vi "Occupancy Grid Drawing.vi"() -> ()   [LabVIEW 2014]
panel:
  out "Occupancy Grid Drawing":dbl[][](graph)
  out "Output Occupancy Grid":dbl[][](array[numeric])
  out "Intermediate Value Array":dbl[][](array[numeric])
  in  "Particle Points":dbl[][](array[numeric])
  # "CM(X), CM(Y), Left X, Right X"
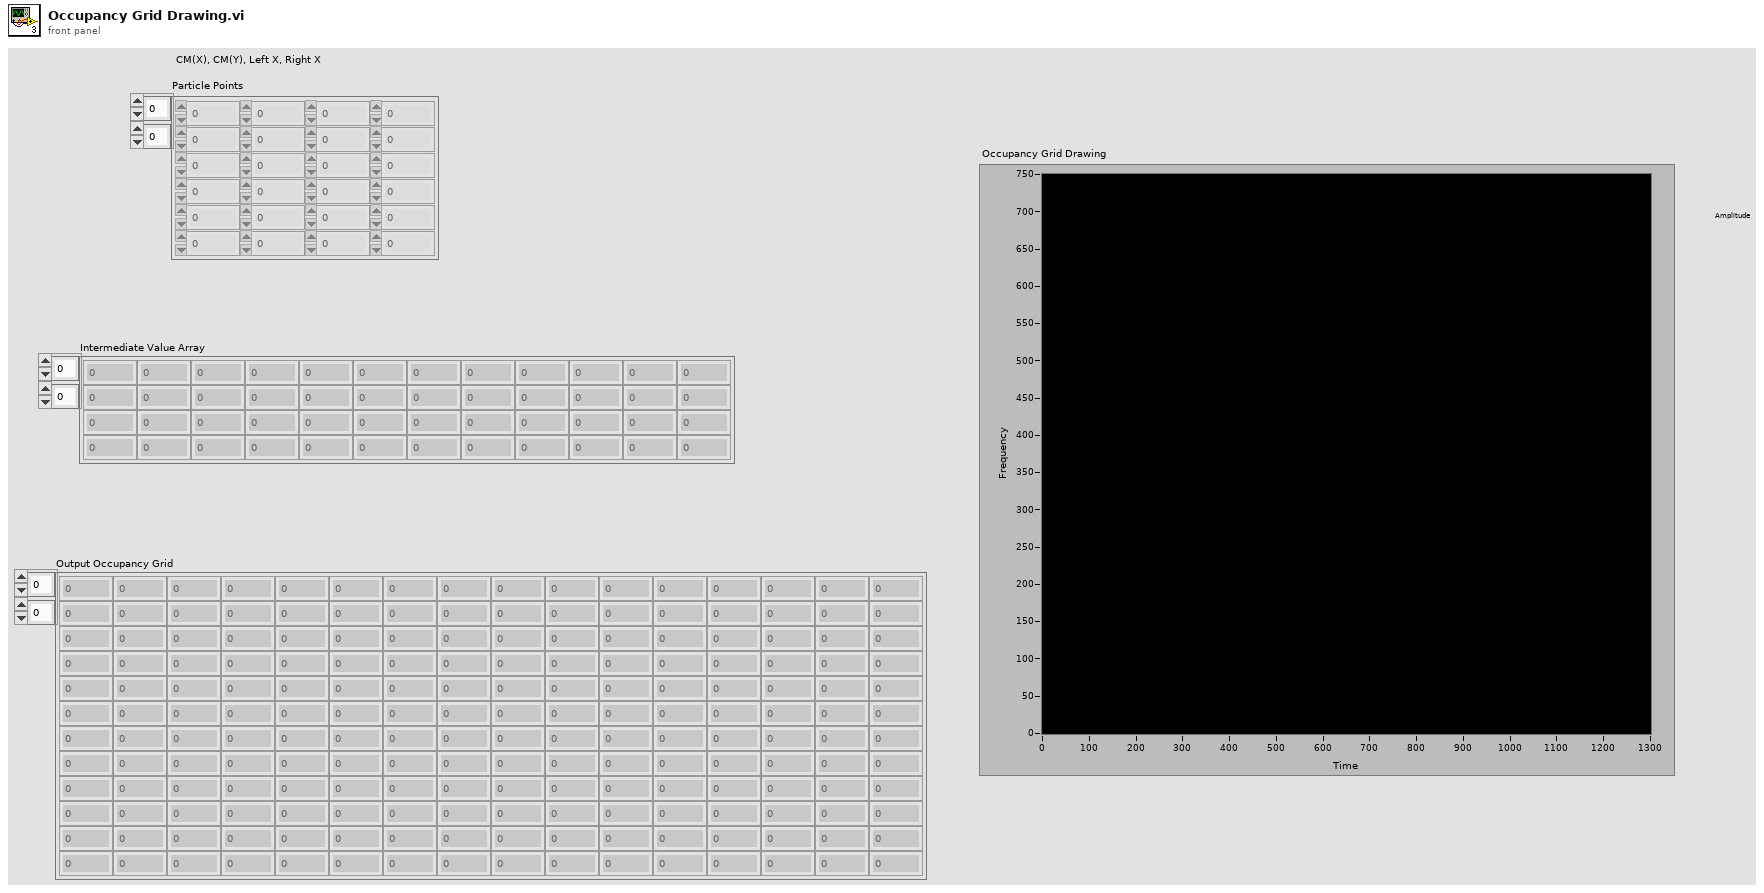
[diagram p1: front panel]
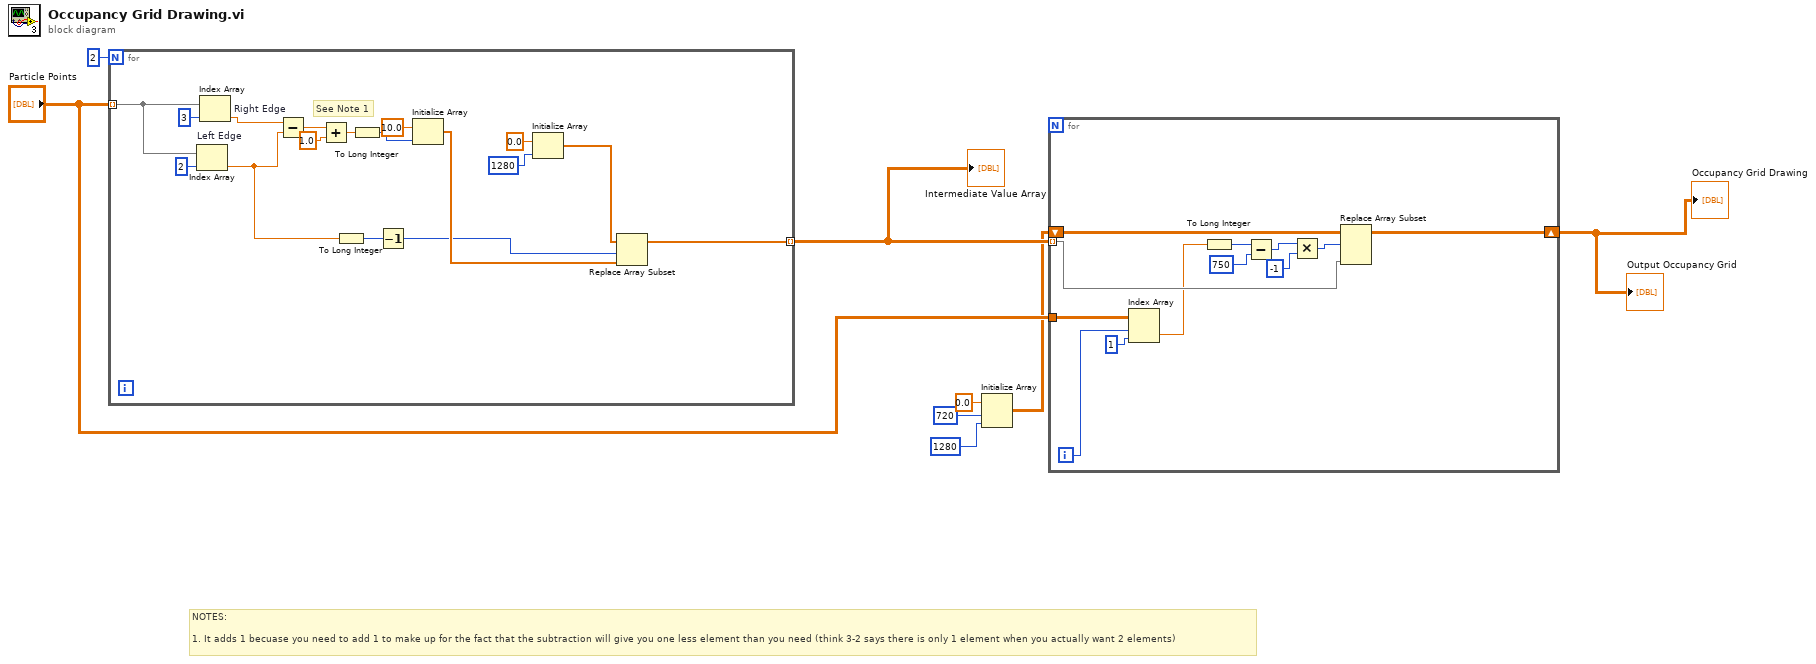
[diagram p0: block diagram]
diagram:
  # "NOTES:\n\n1. It adds 1 becuase you need to add 1 to make up for the fact that the subtraction will give you one less element than you need (think 3-2 says there is only 1 element when you actually want 2 elements)"
  n1 = for {
    N: 2 -> [_]
    tunnel: "Particle Points" -> [w22] mode=indexing
    tunnel: [w12] -> w5 mode=indexing
    # "See Note 1"
    n2 = Index Array "Left Edge"(array=w22, index=2) -> (element=w11:dbl)
    n3 = Index Array "Right Edge"(array=w22, index=3) -> (element=w13:dbl)
    n4 = Subtract(x=w13, y=w11) -> (x-y=w21:dbl)
    n5 = Add(x=w21, y=1.0) -> (x+y=w19:dbl)
    n6 = To Long Integer(number=w11) -> (32bit integer=w10:i32)
    n7 = To Long Integer(number=w19) -> (32bit integer=w17:i32)
    n8 = Decrement(x=w10) -> (x-1=w9:i32)
    n9 = Initialize Array(10.0 ("element"), w17) -> (w15:dbl[])
    n10 = Initialize Array(0.0 ("element"), 1280 ("dimension size")) -> (w14:dbl[])
    n11 = Replace Array Subset(array=w14, new element=w15, index=w9) -> (w12:dbl[])
  }
  "Intermediate Value Array" <- w5
  n12 = Initialize Array(0.0 ("element"), 720 ("dimension size"), 1280 ("dimension size")) -> (w2:dbl[][])
  n13 = for {
    tunnel: w5 -> [w34] mode=indexing
    tunnel: "Particle Points" -> [w37]
    shift-right: [w32] -> w1
    shift-left: w2 -> [w35]
    i -> [w31]
    n14 = Index Array(array=w37, index (row)=w31, index (col)=1 ("disabled index (col)")) -> (element=w33:dbl)
    n15 = To Long Integer(number=w33) -> (32bit integer=w30:i32)
    n16 = Subtract(x=w30, y=750) -> (x-y=w28:i32)
    n17 = Multiply(x=w28, y=-1) -> (x*y=w26:i32)
    n18 = Replace Array Subset(array=w35, new element=w34, index (row)=w26) -> (w32:dbl[][])  [unwired: 1 in]
  }
  "Output Occupancy Grid" <- w1
  "Occupancy Grid Drawing" <- w1
